vi "Wavelength_to_Pixel_Index.vi"(3 "Central Wavelength":dbl=600.0 format="%.2f", 4 "Wavelength for Pixel i":dbl=600.0 format="%.2f", 5 "File Info In":T1={"FilePath"=path "/DATA/Labview Items", "Field (T)"=12.0, "Temperature (K)"=12.0, "X-Axis"=enum."nm", "Center nm"=-1.0, "Current Grating Density"=enum."600", "CCD Parameters"={"Exposure Time (s)"=0.2, "Offset"=0.0, "BkgrdCrct"=FALSE, "Shutter"=FALSE, "Mode"=enum."Regular", "Repetition"=4, "dt or s"=0.0}, "Operation Mode"=enum."NML Data Acquisition", "Exp Index"=3, "Index_repetition"=0, "Index"=0, "Current Detector"=enum."CCD-1024x256"} {"CCD Parameters"."dt or s" format="%#.6f"; "CCD Parameters"."Repetition" min=1; "CCD Parameters"."Offset" format="%#.2f"; "CCD Parameters"."Exposure Time (s)" min=0.02 max=6000.0 format="%#.2f"; "Center nm" format="%.2f"; "Temperature (K)" format="%.2f"; "Field (T)" format="%.2f"}) -> (1 "index (out)":dbl=571.2504622529284 format="%.4f")   [LabVIEW 2024]
uses:
  Globals and TypeDefs/Type Definitions.llb/FileInfoParameter.ctt
  Globals and TypeDefs/Type Definitions.llb/Wavelength Unit.ctt
  Globals and TypeDefs/Type Definitions.llb/McPherson Grating Density.ctl
  Globals and TypeDefs/Type Definitions.llb/CCDParameter.ctt
  Globals and TypeDefs/Type Definitions.llb/OperationMode.ctt
  Globals and TypeDefs/Type Definitions.llb/ListOfDetectors.ctt
panel:
  out "Detector Pixel Distance":dbl=27.0 format="%.2f"
  out "Spectrometer Mirror angle":dbl=21.18 format="%.2f"
  out "Spectrometer Focal length":dbl=750.0 format="%.1f"
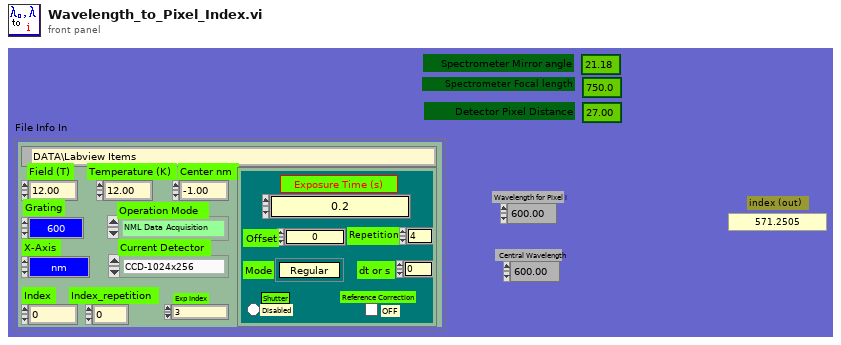
[diagram p1: front panel]
types:
  T1 = typedef "FileInfoParameter.ctt" = cluster{"FilePath":path, "Field (T)":dbl, "Temperature (K)":dbl, "X-Axis":T2, "Center nm":dbl, "Current Grating Density":T3, "CCD Parameters":T4, "Operation Mode":T5, "Exp Index":u32, "Index_repetition":u16, "Index":u16, "Current Detector":T6}
  T2 = typedef "Wavelength Unit.ctt" = enum8{"Point", "nm", "eV", "meV", "cm_1"}
  T3 = typedef "McPherson Grating Density.ctl" = enum8{"150", "300", "600", "1200", "1800"}
  T4 = typedef "CCDParameter.ctt" = cluster{"Exposure Time (s)":dbl, "Offset":dbl, "BkgrdCrct":bool, "Shutter":bool, "Mode":enum8{"Regular", "OverExp Cor", "SpikeRemove", "ForCalibration"}, "Repetition":u16, "dt or s":dbl}
  T5 = typedef "OperationMode.ctt" = enum16{"Standby", "CCD Single Shot", "CCD Sequence Shots", "CCD Custom Shots", "CCD Reference Shot", "Step Scanning ", "Time Scanning", "NML Data Acquisition"}
  T6 = typedef "ListOfDetectors.ctt" = enum8{"CCD-1024x256", "InGaAs PDA-1024x1", "CCD-1340x400", "Ge Single Channel", "Si Single Channel", "PMT Single Channel"}
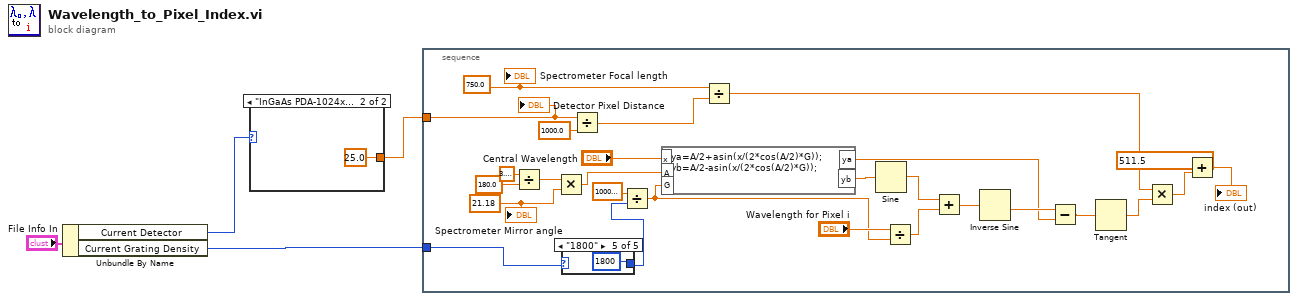
[diagram p0: block diagram]
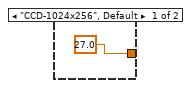
[diagram p2: hidden frame]
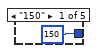
[diagram p3: hidden frame]
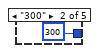
[diagram p4: hidden frame]
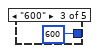
[diagram p5: hidden frame]
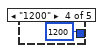
[diagram p6: hidden frame]
diagram:
  n1 = Unbundle By Name("File Info In") -> ("Current Detector"=w4:T6, "Current Grating Density"=w1:T3)
  n2 = case shown="\"InGaAs PDA-1024x1\"" w4 {
    tunnel: [27.0 ("x") 25.0 ("x")] -> w3
    frame "CCD-1024x256", Default {
    }
    frame "InGaAs PDA-1024x1" {
    }
  }
  n3 = stacked-sequence {
    tunnel: w3 -> [w8]
    tunnel: w1 -> [w7]
    frame #0 {
      w30 = 21.18 ("Detector Pixel Distance")
      w24 = 750.0 ("Detector Pixel Distance")
      n4 = Divide(x=3.141592653589793, y=180.0) -> (x/y=w28:dbl)
      n5 = Multiply(x=w28, y=w30) -> (x*y=w29:dbl)
      n6 = case shown="\"1800\"" w7 {
        tunnel: [150 300 600 1200 1800] -> w26
        frame "150" {
        }
        frame "300" {
        }
        frame "600" {
        }
        frame "1200" {
        }
        frame "1800" {
        }
      }
      n7 = Divide(x=w8, y=1000.0) -> (x/y=w23:dbl)
      n8 = Divide(x=1000000.0, y=w26) -> (x/y=w20:dbl)
      n9 = formula code="ya=A/2+asin(x/(2*cos(A/2)*G));\nyb=A/2-asin(x/(2*cos(A/2)*G));"("x"="Central Wavelength", "A"=w29, "G"=w20) -> ("ya"=w15:dbl, "yb"=w21:dbl)
      n10 = Divide(x=w24, y=w23) -> (x/y=w12:dbl)
      n11 = Sine(x=w21) -> (sin(x)=w19:dbl)
      n12 = Divide(x="Wavelength for Pixel i", y=w20) -> (x/y=w18:dbl)
      n13 = Add(x=w19, y=w18) -> (x+y=w17:dbl)
      n14 = Inverse Sine(1:w17) -> (0:w16:dbl)
      n15 = Subtract(x=w16, y=w15) -> (x-y=w14:dbl)
      n16 = Tangent(1:w14) -> (0:w13:dbl)
      n17 = Multiply(x=w12, y=w13) -> (x*y=w10:dbl)
      n18 = Add(x=511.5, y=w10) -> (x+y=→"index (out)":dbl)
      "Spectrometer Focal length" <- w24
      "Spectrometer Mirror angle" <- w30
      "Detector Pixel Distance" <- w8
    }
  }
